vi "Parameter Ring Chooser.vi"(8 "error in (no error)":errorcluster, 11 "Generic Digital Multi Meter in":refnum<class "Generic Digital Multi Meter.lvclass">) -> (0 "error out":errorcluster, 3 "Generic Digital Multi Meter out":refnum<class "Generic Digital Multi Meter.lvclass">)   [LabVIEW 2014, in "Generic Digital Multi Meter.lvlib" / "Generic Digital Multi Meter.lvclass"]
uses:
  Generic Digital Multi Meter.lvclass
panel:
  in  "Measurement Function (0: DC Volts)":u16(ring) items=["DC Volts", "AC Volts", "DC Current", "AC Current", "2-Wire Resistance", "4-Wire Resistance", "Frequency", "AC and DC rms Current", "AC and DC rms Volts", "Continuity", "Diode"]
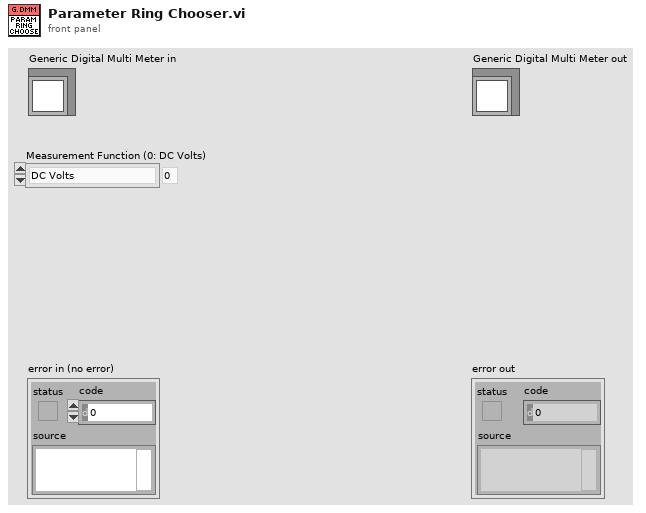
[diagram p1: front panel]
types:
  T1 = typedef "LVStringsAndValuesArrayTypeDef_U16.ctl" = cluster{"String":string, "Value":u16}[]
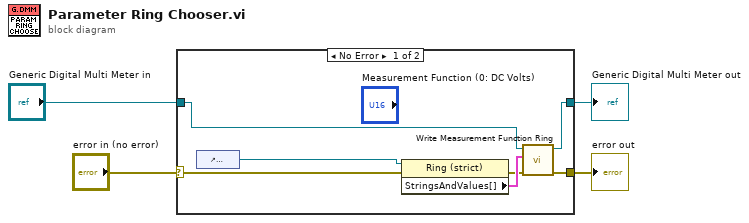
[diagram p0: block diagram]
diagram:
  n1 = case shown="No Error" "error in (no error)" {
    selector: "error in (no error)" -> [w6 w13]
    tunnel: [w9 w13] -> w3
    tunnel: [w10 w12] -> w1
    tunnel: "Generic Digital Multi Meter in" -> [w11 w12]
    frame No Error {
      n2 = control-ref of="Measurement Function (0: DC Volts)"() -> (w8:refnum<vi>)
      n3 = property class="Ring (strict)"(reference=w8, error in=w6) -> (error out=w5:errorcluster, "StringsAndValues[]"=w7:T1)  [unwired: 1 out]
      n4 = call-dynamic "Write Measurement Function Ring.vi"("error in (no error)"=w5, "Strings And Values []"=w7, "Generic Digital Multi Meter in"=w11) -> ("error out"=w9:errorcluster, "Generic Digital Multi Meter out"=w10:refnum<class "Generic Digital Multi Meter.lvclass">)  [unwired: 7 in]
    }
    frame Error {
    }
  }
  "error out" <- w3
  "Generic Digital Multi Meter out" <- w1
